vi "GV-ConvRangeScale.vi"(10 "RangeL":dbl, 11 "RangeH":dbl) -> (2 "Offset":dbl, 3 "Gain":dbl)   [LabVIEW 2020, in "Sgraph_lib_V1.lvlib" / "Gviewer.lvclass"]
doc: "Convert RangeH and RangeL into Gain and Offset for Graph display"
uses:
  Gviewer.lvclass
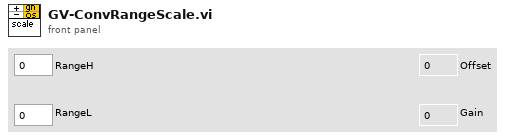
[diagram p1: front panel]
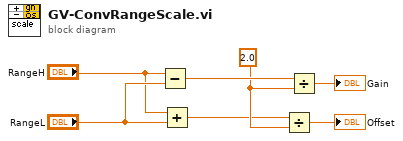
[diagram p0: block diagram]
diagram:
  w3 = 2.0 ("x")
  n1 = Subtract(x="RangeH", y="RangeL") -> (x-y=w4:dbl)
  n2 = Add(x="RangeH", y="RangeL") -> (x+y=w1:dbl)
  n3 = Divide(x=w1, y=w3) -> (x/y=→"Offset":dbl)
  n4 = Divide(x=w4, y=w3) -> (x/y=→"Gain":dbl)
